vi "外观 1.vi"(0 "Data In":T5 caption="数据输入", 2 "Display State In":T3 caption="显示状态输入", 3 "Container State":T4 caption="容器状态") -> (6 "Data Out":T5 caption="数据输出", 7 "Display State Out":T3 caption="显示状态输出", 8 "Action":T2 caption="动作")   [LabVIEW 2016, in "24H周期设置.xctl"]
uses:
  <vilib>/_xctls/Container State.ctl
  <vilib>/_xctls/Action.ctl
  <vilib>/Utility/miscctls.llb/LVPointTypeDef.ctl
  <vilib>/_xctls/XControlSupport.lvlib
panel:
  in  "簇":T1
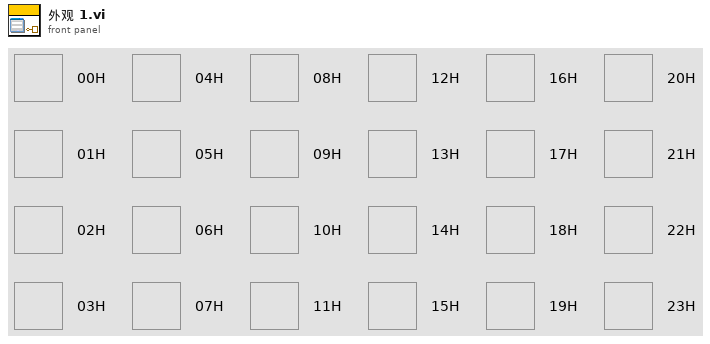
[diagram p1: front panel]
types:
  T1 = cluster{"00H":bool, "01H":bool, "02H":bool, "03H":bool, "04H":bool, "05H":bool, "06H":bool, "07H":bool, "08H":bool, "09H":bool, "10H":bool, "11H":bool, "12H":bool, "13H":bool, "14H":bool, "15H":bool, "16H":bool, "17H":bool, "18H":bool, "19H":bool, "20H":bool, "21H":bool, "22H":bool, "23H":bool}
  T2 = typedef "XControlSupport.lvlib/Action.ctl" = cluster{"Data Changed?":bool, "State Changed?":bool, "Action Name":string}
  T3 = typedef "24H周期设置.xctl/状态 1.ctl" = cluster{"Numeric":dbl}
  T4 = typedef "XControlSupport.lvlib/Container State.ctl" = cluster{"Indicator?":bool, "Run Mode?":bool, " Refnum":refnum<vi>}
  T5 = typedef "24H周期设置.xctl/数据 1.ctl" = cluster{"00H":bool, "01H":bool, "02H":bool, "03H":bool, "04H":bool, "05H":bool, "06H":bool, "07H":bool, "08H":bool, "09H":bool, "10H":bool, "11H":bool, "12H":bool, "13H":bool, "14H":bool, "15H":bool, "16H":bool, "17H":bool, "18H":bool, "19H":bool, "20H":bool, "21H":bool, "22H":bool, "23H":bool}
  T6 = typedef "LVPointTypeDef.ctl" = cluster{"Horizontal":i16, "Vertical":i16}
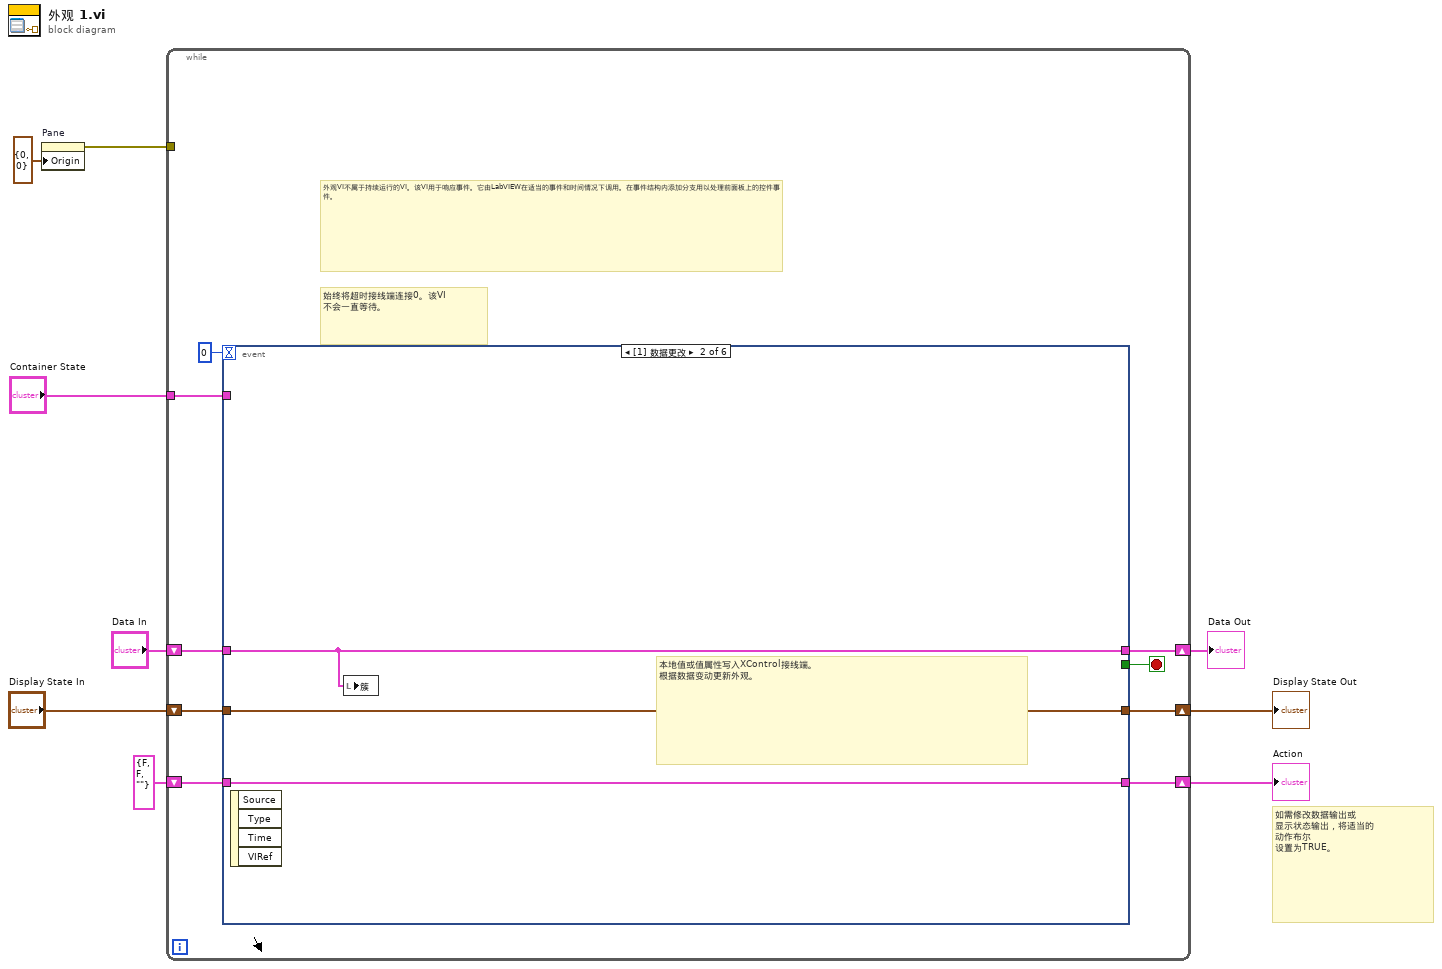
[diagram p0: block diagram]
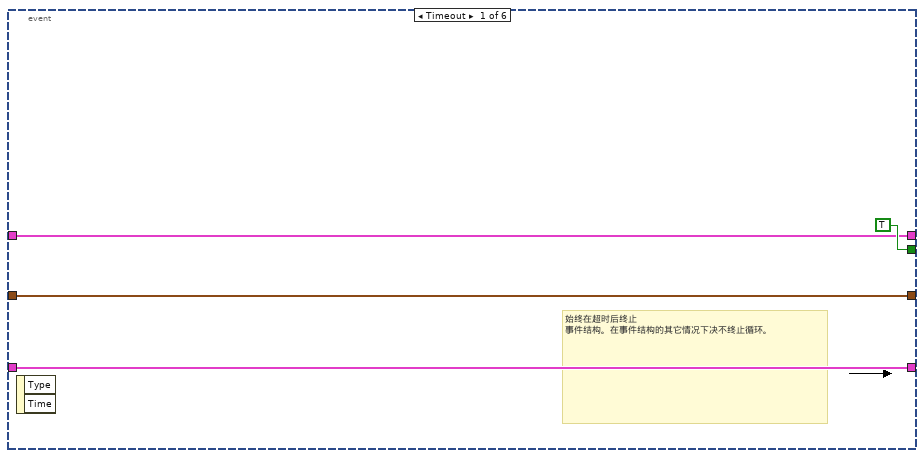
[diagram p2: hidden frame]
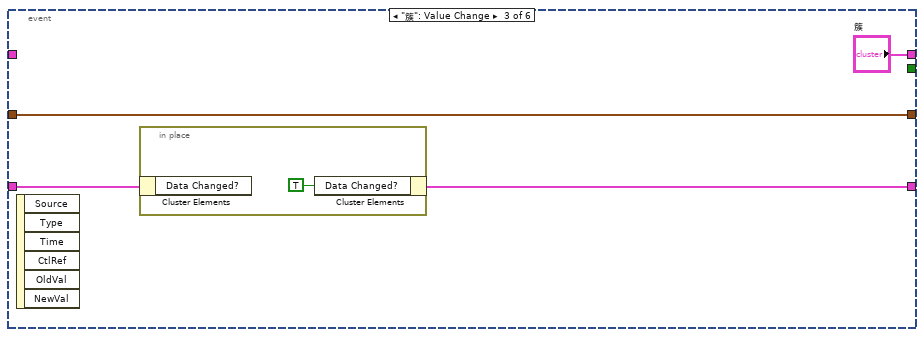
[diagram p3: hidden frame]
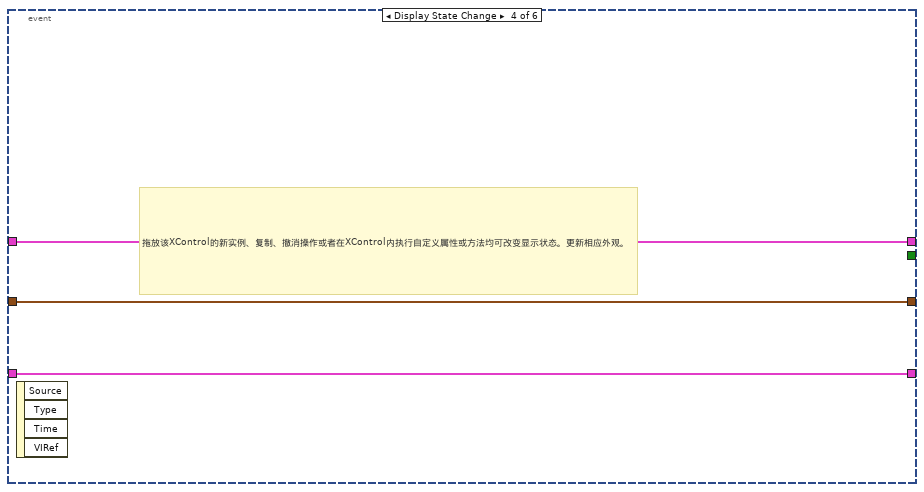
[diagram p4: hidden frame]
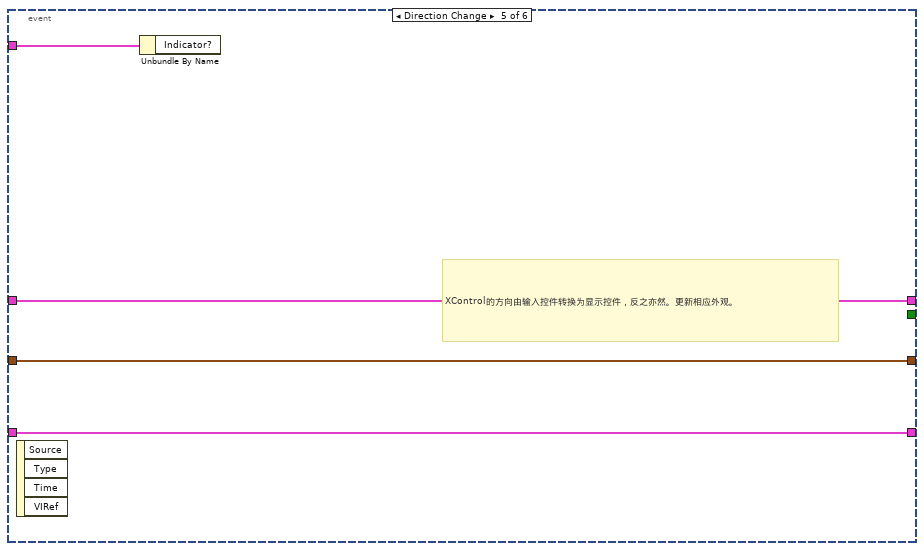
[diagram p5: hidden frame]
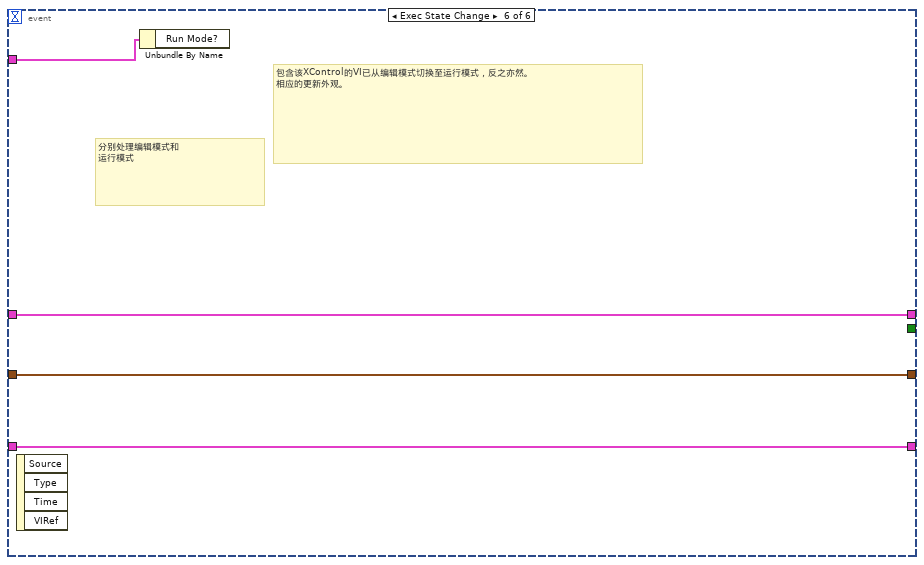
[diagram p6: hidden frame]
diagram:
  # "如需修改数据输出或\n显示状态输出，将适当的\n动作布尔\n设置为TRUE。"
  n1 = property on="Pane" class="Pane"("Origin"=T6 {"Horizontal"=0, "Vertical"=0} ("原点")) -> (error out=w1:errorcluster)  [unwired: 2 in, 1 out]
  n2 = while {
    shift-right: [w17] -> w6
    shift-left: "Display State In" -> [w18]
    tunnel: "Container State" -> [w14]
    shift-right: [w12] -> w9
    shift-left: "Data In" -> [w13]
    shift-right: [w10] -> w4
    shift-left: T2 {"Data Changed?"=FALSE, "State Changed?"=FALSE, "Action Name"=""} ("Action") -> [w11]
    tunnel: w1 -> [_]
    stop <- w16 stop-if-true
    # "外观VI不属于持续运行的VI。该VI用于响应事件。它由LabVIEW在适当的事件和时间情况下调用。在事件结构内添加分支用以处理前面板上的控件事件。"
    # "始终将超时接线端连接0。该VI\n不会一直等待。"
    n3 = event shown="[1] 数据更改" {
      selector: _ -> [_ _ _ _ _ _]
      dyn-events: _ -> [_ _ _ _ _ _]
      timeout: 0 -> [_ _ _ _ _ _]
      tunnel: w18 -> [w20 w25 w29 w33 w36 w40]
      tunnel: [w20 w25 w29 w33 w36 w40] -> w17
      tunnel: [TRUE _ _ _ _ _] -> w16
      tunnel: w14 -> [_ _ _ _ w37 w41]
      tunnel: w13 -> [w19 w23 _ w32 w35 w39]
      tunnel: [w19 w23 "簇" w32 w35 w39] -> w12
      tunnel: [w21 w24 w26 w31 w34 w38] -> w10
      tunnel: w11 -> [w21 w24 w27 w31 w34 w38]
      event Timeout {
        # "始终在超时后终止\n事件结构。在事件结构的其它情况下决不终止循环。"
        n4 = event-data() -> ()  [unwired: 1 in, 2 out]
      }
      event Data Change {
        # "本地值或值属性写入XControl接线端。\n根据数据变动更新外观。"
        n5 = event-data() -> ()  [unwired: 1 in, 4 out]
        n6 = local write "簇"(w23) -> ()
      }
      event "簇": Value Change {
        n7 = event-data() -> ()  [unwired: 1 in, 6 out]
        n8 = in-place {
          n9 = in-place-cluster #1(w27) -> ()  [unwired: 1 out]
          n10 = in-place-cluster #1("Data Changed?"=TRUE) -> (w26:T2)
        }
      }
      event Display State Change {
        # "拖放该XControl的新实例、复制、撤消操作或者在XControl内执行自定义属性或方法均可改变显示状态。更新相应外观。"
        n11 = event-data() -> ()  [unwired: 1 in, 4 out]
      }
      event Direction Change {
        # "XControl的方向由输入控件转换为显示控件，反之亦然。更新相应外观。"
        n12 = event-data() -> ()  [unwired: 1 in, 4 out]
        n13 = Unbundle By Name(w37) -> ()  [unwired: 1 out]
      }
      event Exec State Change {
        # "包含该XControl的VI已从编辑模式切换至运行模式，反之亦然。\n相应的更新外观。"
        # "分别处理编辑模式和\n运行模式"
        n14 = event-data() -> ()  [unwired: 1 in, 4 out]
        n15 = Unbundle By Name(w41) -> ()  [unwired: 1 out]
      }
    }
  }
  "Display State Out" <- w6
  "Data Out" <- w9
  "Action" <- w4
